vi "teste-Image-2.vi"() -> ()   [LabVIEW 2014]
panel:
  out "size(s) 3":i32=5760000
  out "image":u8[](array[numeric])
  out "size(s) 2":i32=1600
  out "size(s)":i32[](array[numeric])=[1200, 1600]
  out "Waveform Graph":u8[](graph)=[0, 0, 0, 0, 0, 0, 0, 0, 0, 0, 0, 0, 0, 0, 0, 0, 0, 0, 0, 0, 0, 0, 0, 0, 0, 0, 0, 0, 0, 0, 0, 0, 0, 0, 0, 0, 0, 0, 0, 0, 0, 0, 0, 0, 0, 0, 0, 0, 0, 0, 0, 0, 0, 0, 0, 0, 0, 0, 0, 0, 0, 0, 0, 0, 0, 0, 0, 0, 0, 0, 0, 0, 0, 0, 0, 0, 0, 0, 0, 0, 0, 0, 0, 0, 0, 0, 0, 0, 0, 0, 0, 0, 0, 0, 0, 0, 0, 0, 0, 0, 0, 0, 0, 0, 0, 0, 0, 0, 0, 0, 0, 0, 0, 0, 0, 0, 0, 0, 0, 0, 0, 0, 0, 0, 0, 0, 0, 0, 0, 0, 0, 0, 0, 0, 0, 0, 0, 0, 0, 0, 0, 0, 0, 0, 0, 0, 0, 0, 0, 0, 0, 0, 0, 0, 0, 0, 0, 0, 0, 0, 0, 0, 0, 0, 0, 0, 0, 0, 0, 0, 0, 0, 0, 0, 0, 0, 0, 0, 0, 0, 0, 0, 0, 0, 2, 2, 1, 0, 0, 0, 0, 1, 0, 0, 1, 1, 0, 0, 1, 2, 0, 0, 0, 0, 0, 0, 0, 0, 0, 0, 0, 0, 0, 0, 0, 0, 0, 0, 0, 0, 0, 0, 0, 0, 1, 1, 1, 1, 1, 1, 1, 1, 1, 1, 3, 5, 3, 1, 1, 3, 0, 0, 0, 0, 0, 0, 0, 0, 0, 0, 0, 0, 0, 0, 0, 0, 0, 0, 0, 0, 0, 0, 0, 0, 0, 0, 0, 0, 0, 0, 0, 0, 0, 3, 4, 0, 1, 4, 5, 3, 4, 4, 4, 1, 0, 0, 0, 0, 0, 0, 0, 0, 0, 0, 0, 0, 0, 0, 0, 0, 0, 0, 0, 0, 0, 0, 0, 0, 0, 0, 0, 0, 0, 0, 0, 0, 0, 0, 0, 0, 0, 0, 0, 0, 0, 0, 0, 0, 0, 0, 0, 0, 0, 0, 0, 0, 0, 0, 0, 0, 0, 0, 0, 0, 0, 0, 0, 0, 0, 0, 0, 0, 2, 4, 7, 5, 4, 1, 5, 5, 4, 2, 4, 2, 7, 9, 13, 10, 1, 0, 0, 0, 0, 0, 0, 0, 0, 1, 2, 2, 0, 0, 1, 3, 2, 4, 3, 3, 4, 4, 4, 4, 7, 8, 9, 5, 5, 5, 6, 3, 2, 1, 1, 3, 4, 6, 10, 11, 11, 9, 8, 12, 16, 17, 13, 10, 28, 28, 18, 26, 13, 26, 14, 7, 11, 9, 11, 15, 13, 15, 16, 34, 10, 10, 13, 8, 10, 11, 14, 34, 11, 12, 9, 9, 8, 7, 9, 13, 10, 14, 9, 10, 6, 3, 5, 3, 4, 4, 10, 5, 7, 8, 13, 9, 10, 11, 10, 8, 5, 4, 5, 4, 0, 0, 1, 1, 0, 0, 0, 0, 0, 1, 1, 1, 1, 1, 1, 1, 2, 1, 1, 1, 1, 1, 1, 2, 0, 0, 0, 0, 0, 0, 0, 0, 2, 2, 2, 2, 1, 0, 0, 1, 5, 2, 1, 1, 4, 5, 3, 1, 4, 1, 1, 3, 5, 3, 4, 5, 8, 8, 11, 13, 9, 6, 9, 15, 9, 16, 18, 20, 24, 49, 40, 33, 56, 47, 28, 46, 33, 58, 62, 66, 72, 56, 53, 35, 40, 46, 63, 73, 83, 83, 80, 79, 78, 75, 75, 75, 75, 76, 66, 71, 71, 65, 76, 79, 82, 86, 87, 90, 91, 91, 91, 92, 98, 95, 95, 99, 99, 97, 99, 102, 98, 101, 102, 100, 100, 101, 100, 97, 100, 99, 99, 101, 103, 103, 101, 98, 98, 98, 99, 97, 99, 97, 97, 97, 99, 97, 94, 93, 94, 95, 96, 95, 90, 91, 93, 93, 91, 89, 88, 88, 85, 86, 85, 83, 81, 80, 81, 81, 85, 83, 83, 85, 84, 81, 77, 80, 86, 84, 80, 77, 78, 78, 79, 74, 67, 41, 40, 39, 56, 42, 45, 44, 47, 47, 54, 64, 71, 73, 74, 74, 68, 54, 66, 54, 65, 69, 55, 69, 63, 66, 74, 81, 77, 78, 84, 91, 96, 99, 98, 98, 96, 95, 94, 94, 96, 98, 98, 100, 101, 101, 103, 103, 106, 106, 109, 109, 111, 113, 114, 114, 116, 114, 115, 113, 114, 113, 114, 115, 115, 116, 117, 120, 120, 120, 121, 121, 120, 120, 123, 123, 125, 125, 126, 126, 127, 127, 129, 130, 131, 131, 134, 134, 136, 136, 136, 136, 136, 135, 137, 135, 134, 132, 131, 131, 131, 130, 130, 129, 129, 128, 128, 128, 128, 128, 126, 126, 125, 125, 125, 126, 128, 128, 130, 130, 130, 130, 128, 128, 126, 125, 125, 125, 125, 125, 125, 124, 123, 122, 122, 122, 124, 122, 124, 121, 121, 120, 120, 120, 121, 121, 120, 119, 118, 118, 118, 118, 115, 115, 115, 116, 116, 115, 114, 113, 104, 103, 104, 103, 99, 98, 98, 97, 96, 94, 93, 90, 90, 90, 91, 90, 86, 86, 84, 75, 76, 79, 53, 39, 41, 33, 27, 24, 21, 16, 14, 14, 22, 25, 9, 7, 6, 4, 15, 4, 3, 1, 1, 1, 2, 4, 3, 3, 8, 12, 13, 7, 4, 4, 6, 4, 4, 6, 7, 3, 5, 3, 4, 5, 7, 4, 6, 15, 13, 37, 19, 8, 8, 1, 1, 4, 4, 10, 15, 12, 8, 12, 13, 26, 36, 35, 42, 49, 31, 38, 35, 41, 44, 73, 54, 54, 57, 54, 55, 72, 64, 78, 69, 73, 77, 78, 73, 67, 71, 72, 68, 72, 81, 85, 87, 87, 85, 87, 88, 90, 89, 90, 91, 93, 93, 91, 89, 85, 76, 74, 69, 81, 76, 68, 63, 86, 80, 85, 84, 82, 83, 86, 85, 79, 73, 68, 80, 61, 46, 41, 49, 43, 45, 59, 48, 53, 59, 54, 58, 72, 56, 71, 71, 61, 71, 60, 49, 50, 45, 27, 20, 23, 13, 16, 28, 13, 8, 11, 14, 10, 4, 3, 1, 2, 1, 1, 1, 0, 1, 0, 0, 0, 0, 0, 0, 0, 0, 0, 0, 0, 0, 0, 0, 0, 0, 0, 0, 0, 0, 0, 0, 0, 0, 0, 0, 0, 0, 0, 0, 0, 0, 0, 0, 0, 0, 0, 0, 0, 0, 0, 1, 1, 15, 7, 1, 1, 4, 2, 4, 5, 4, 5, 4, 4, 2, 2, 1, 0, 0, 1, 2, 3, 5, 5, 6, 6, 3, 4, 4, 3, 3, 7, 6, 3, 3, 3, 3, 3, 3, 3, 3, 3, 7, 3, 8, 6, 41, 15, 12, 39, 26, 18, 12, 10, 8, 3, 1, 5, 21, 4, 3, 9, 5, 10, 15, 6, 7, 5, 4, 3, 2, 1, 1, 3, 1, 3, 4, 4, 1, 1, 5, 1, 1, 1, 1, 1, 1, 1, 1, 1, 1, 2, 3, 2, 1, 1, 2, 4, 2, 2, 2, 1, 1, 3, 10, 15, 4, 1, 0, 0, 3, 4, 2, 0, 0, 0, 0, 0, 0, 0, 0, 0, 0, 0, 0, 0, 0, 0, 0, 0, 0, 0, 0, 0, 0, 0, 0, 0, 0, 0, 0, 0, 0, 0, 0, 0, 0, 0, 0, 0, 0, 0, 0, 0, 0, 0, 0, 0, 0, 0, 0, 0, 0, 0, 0, 0, 0, 0, 0, 0, 1, 0, 0, 0, 0, 0, 0, 1, 0, 0, 0, 0, 0, 0, 0, 0, 0, 0, 0, 0, 0, 0, 0, 0, 0, 0, 0, 0, 0, 0, 0, 0, 0, 0, 0, 0, 0, 0, 0, 0, 0, 0, 0, 0, 0, 0, 0, 0, 0, 0, 0, 0, 0, 0, 0, 0, 0, 0, 0, 0, 0, 0, 0, 0, 0, 0, 0, 0, 0, 0, 0, 0, 0, 0, 0, 0, 0, 0, 0, 0, 0, 0, 0, 0, 0, 0, 0, 0, 0, 0, 0, 0, 0, 0, 0, 0, 0, 0, 0, 0, 0, 0, 0, 0, 0, 0, 0, 0, 0, 0, 0, 0, 0, 0, 0, 0, 0, 0, 0, 0, 0, 0, 0, 0, 0, 0, 0, 0, 0, 0, 0, 0, 0, 0, 0, 0, 0, 0, 0, 0, 0, 0, 0, 0, 0, 0, 0, 0, 0, 0, 0, 0, 0, 0, 0, 0, 0, 0, 0, 0, 0, 0, 0, 0, 0, 0, 0, 0, 0, 0, 0, 0, 0, 0, 0, 0, 0, 0, 0, 0, 0, 0, 0, 0, 0, 0, 0, 0, 0, 0, 0, 0, 0, 0, 0, 0, 0, 0, 0, 0, 0, 0, 0, 0, 0, 0, 0, 0, 0, 0, 0, 0, 0, 0, 0, 0, 0, 0, 0, 0, 0, 0, 0, 0, 0, 0, 0, 0, 0, 0, 0, 0, 0, 0, 0, 0, 0, 0, 0, 0, 1, 0, 0, 0, 0, 0, 0, 1, 0, 0, 0, 0, 0, 0, 0, 0, 0, 0, 0, 0, 0, 0, 0, 0, 0, 0, 0, 0, 0, 0, 0, 0, 0, 0, 0, 0, 0, 0, 0, 0, 0, 0, 0, 0, 0, 0, 0, 0, 0, 0, 0, 0, 0, 0, 0, 0, 0, 0, 0, 0, 0, 0, 0, 0, 0, 0, 0, 0, 0, 0, 0, 0, 0, 0, 0, 0, 0, 0, 0, 0, 0, 0, 0, 0, 0, 0, 0, 0, 0, 0, 0, 0, 0, 0, 0, 0, 0, 0, 0, 0, 0, 0, 0, 0, 0, 0, 0, 0, 0, 0, 0, 0, 0, 0, 2, 4, 4, 2, 0, 0, 0, 0, 0, 0, 0, 0, 0, 0, 0, 0, 0, 0, 0, 0, 0, 0, 0, 0, 0, 0, 0, 0, 0, 0]
  out "2D Picture":picture
  out "subarray":u8[](array[numeric])=[0, 0, 0, 0, 0, 0, 0, 0, 0, 0, 0, 0, 0, 0, 0, 0, 0, 0, 0, 0, 0, 0, 0, 0, 0, 0, 0, 0, 0, 0, 0, 0, 0, 0, 0, 0, 0, 0, 0, 0, 0, 0, 0, 0, 0, 0, 0, 0, 0, 0, 0, 0, 0, 0, 0, 0, 0, 0, 0, 0, 0, 0, 0, 0, 0, 0, 0, 0, 0, 0, 0, 0, 0, 0, 0, 0, 0, 0, 0, 0, 0, 0, 0, 0, 0, 0, 0, 0, 0, 0, 0, 0, 0, 0, 0, 0, 0, 0, 0, 0, 0, 0, 0, 0, 0, 0, 0, 0, 0, 0, 0, 0, 0, 0, 0, 0, 0, 0, 0, 0, 0, 0, 0, 0, 0, 0, 0, 0, 0, 0, 0, 0, 0, 0, 0, 0, 0, 0, 0, 0, 0, 0, 0, 0, 0, 0, 0, 0, 0, 0, 0, 0, 0, 0, 0, 0, 0, 0, 0, 0, 0, 0, 0, 0, 0, 0, 0, 0, 0, 0, 0, 0, 0, 0, 0, 0, 0, 0, 0, 0, 0, 0, 0, 0, 2, 2, 1, 0, 0, 0, 0, 1, 0, 0, 1, 1, 0, 0, 1, 2, 0, 0, 0, 0, 0, 0, 0, 0, 0, 0, 0, 0, 0, 0, 0, 0, 0, 0, 0, 0, 0, 0, 0, 0, 1, 1, 1, 1, 1, 1, 1, 1, 1, 1, 3, 5, 3, 1, 1, 3, 0, 0, 0, 0, 0, 0, 0, 0, 0, 0, 0, 0, 0, 0, 0, 0, 0, 0, 0, 0, 0, 0, 0, 0, 0, 0, 0, 0, 0, 0, 0, 0, 0, 3, 4, 0, 1, 4, 5, 3, 4, 4, 4, 1, 0, 0, 0, 0, 0, 0, 0, 0, 0, 0, 0, 0, 0, 0, 0, 0, 0, 0, 0, 0, 0, 0, 0, 0, 0, 0, 0, 0, 0, 0, 0, 0, 0, 0, 0, 0, 0, 0, 0, 0, 0, 0, 0, 0, 0, 0, 0, 0, 0, 0, 0, 0, 0, 0, 0, 0, 0, 0, 0, 0, 0, 0, 0, 0, 0, 0, 0, 0, 2, 4, 7, 5, 4, 1, 5, 5, 4, 2, 4, 2, 7, 9, 13, 10, 1, 0, 0, 0, 0, 0, 0, 0, 0, 1, 2, 2, 0, 0, 1, 3, 2, 4, 3, 3, 4, 4, 4, 4, 7, 8, 9, 5, 5, 5, 6, 3, 2, 1, 1, 3, 4, 6, 10, 11, 11, 9, 8, 12, 16, 17, 13, 10, 28, 28, 18, 26, 13, 26, 14, 7, 11, 9, 11, 15, 13, 15, 16, 34, 10, 10, 13, 8, 10, 11, 14, 34, 11, 12, 9, 9, 8, 7, 9, 13, 10, 14, 9, 10, 6, 3, 5, 3, 4, 4, 10, 5, 7, 8, 13, 9, 10, 11, 10, 8, 5, 4, 5, 4, 0, 0, 1, 1, 0, 0, 0, 0, 0, 1, 1, 1, 1, 1, 1, 1, 2, 1, 1, 1, 1, 1, 1, 2, 0, 0, 0, 0, 0, 0, 0, 0, 2, 2, 2, 2, 1, 0, 0, 1, 5, 2, 1, 1, 4, 5, 3, 1, 4, 1, 1, 3, 5, 3, 4, 5, 8, 8, 11, 13, 9, 6, 9, 15, 9, 16, 18, 20, 24, 49, 40, 33, 56, 47, 28, 46, 33, 58, 62, 66, 72, 56, 53, 35, 40, 46, 63, 73, 83, 83, 80, 79, 78, 75, 75, 75, 75, 76, 66, 71, 71, 65, 76, 79, 82, 86, 87, 90, 91, 91, 91, 92, 98, 95, 95, 99, 99, 97, 99, 102, 98, 101, 102, 100, 100, 101, 100, 97, 100, 99, 99, 101, 103, 103, 101, 98, 98, 98, 99, 97, 99, 97, 97, 97, 99, 97, 94, 93, 94, 95, 96, 95, 90, 91, 93, 93, 91, 89, 88, 88, 85, 86, 85, 83, 81, 80, 81, 81, 85, 83, 83, 85, 84, 81, 77, 80, 86, 84, 80, 77, 78, 78, 79, 74, 67, 41, 40, 39, 56, 42, 45, 44, 47, 47, 54, 64, 71, 73, 74, 74, 68, 54, 66, 54, 65, 69, 55, 69, 63, 66, 74, 81, 77, 78, 84, 91, 96, 99, 98, 98, 96, 95, 94, 94, 96, 98, 98, 100, 101, 101, 103, 103, 106, 106, 109, 109, 111, 113, 114, 114, 116, 114, 115, 113, 114, 113, 114, 115, 115, 116, 117, 120, 120, 120, 121, 121, 120, 120, 123, 123, 125, 125, 126, 126, 127, 127, 129, 130, 131, 131, 134, 134, 136, 136, 136, 136, 136, 135, 137, 135, 134, 132, 131, 131, 131, 130, 130, 129, 129, 128, 128, 128, 128, 128, 126, 126, 125, 125, 125, 126, 128, 128, 130, 130, 130, 130, 128, 128, 126, 125, 125, 125, 125, 125, 125, 124, 123, 122, 122, 122, 124, 122, 124, 121, 121, 120, 120, 120, 121, 121, 120, 119, 118, 118, 118, 118, 115, 115, 115, 116, 116, 115, 114, 113, 104, 103, 104, 103, 99, 98, 98, 97, 96, 94, 93, 90, 90, 90, 91, 90, 86, 86, 84, 75, 76, 79, 53, 39, 41, 33, 27, 24, 21, 16, 14, 14, 22, 25, 9, 7, 6, 4, 15, 4, 3, 1, 1, 1, 2, 4, 3, 3, 8, 12, 13, 7, 4, 4, 6, 4, 4, 6, 7, 3, 5, 3, 4, 5, 7, 4, 6, 15, 13, 37, 19, 8, 8, 1, 1, 4, 4, 10, 15, 12, 8, 12, 13, 26, 36, 35, 42, 49, 31, 38, 35, 41, 44, 73, 54, 54, 57, 54, 55, 72, 64, 78, 69, 73, 77, 78, 73, 67, 71, 72, 68, 72, 81, 85, 87, 87, 85, 87, 88, 90, 89, 90, 91, 93, 93, 91, 89, 85, 76, 74, 69, 81, 76, 68, 63, 86, 80, 85, 84, 82, 83, 86, 85, 79, 73, 68, 80, 61, 46, 41, 49, 43, 45, 59, 48, 53, 59, 54, 58, 72, 56, 71, 71, 61, 71, 60, 49, 50, 45, 27, 20, 23, 13, 16, 28, 13, 8, 11, 14, 10, 4, 3, 1, 2, 1, 1, 1, 0, 1, 0, 0, 0, 0, 0, 0, 0, 0, 0, 0, 0, 0, 0, 0, 0, 0, 0, 0, 0, 0, 0, 0, 0, 0, 0, 0, 0, 0, 0, 0, 0, 0, 0, 0, 0, 0, 0, 0, 0, 0, 0, 1, 1, 15, 7, 1, 1, 4, 2, 4, 5, 4, 5, 4, 4, 2, 2, 1, 0, 0, 1, 2, 3, 5, 5, 6, 6, 3, 4, 4, 3, 3, 7, 6, 3, 3, 3, 3, 3, 3, 3, 3, 3, 7, 3, 8, 6, 41, 15, 12, 39, 26, 18, 12, 10, 8, 3, 1, 5, 21, 4, 3, 9, 5, 10, 15, 6, 7, 5, 4, 3, 2, 1, 1, 3, 1, 3, 4, 4, 1, 1, 5, 1, 1, 1, 1, 1, 1, 1, 1, 1, 1, 2, 3, 2, 1, 1, 2, 4, 2, 2, 2, 1, 1, 3, 10, 15, 4, 1, 0, 0, 3, 4, 2, 0, 0, 0, 0, 0, 0, 0, 0, 0, 0, 0, 0, 0, 0, 0, 0, 0, 0, 0, 0, 0, 0, 0, 0, 0, 0, 0, 0, 0, 0, 0, 0, 0, 0, 0, 0, 0, 0, 0, 0, 0, 0, 0, 0, 0, 0, 0, 0, 0, 0, 0, 0, 0, 0, 0, 0, 0, 1, 0, 0, 0, 0, 0, 0, 1, 0, 0, 0, 0, 0, 0, 0, 0, 0, 0, 0, 0, 0, 0, 0, 0, 0, 0, 0, 0, 0, 0, 0, 0, 0, 0, 0, 0, 0, 0, 0, 0, 0, 0, 0, 0, 0, 0, 0, 0, 0, 0, 0, 0, 0, 0, 0, 0, 0, 0, 0, 0, 0, 0, 0, 0, 0, 0, 0, 0, 0, 0, 0, 0, 0, 0, 0, 0, 0, 0, 0, 0, 0, 0, 0, 0, 0, 0, 0, 0, 0, 0, 0, 0, 0, 0, 0, 0, 0, 0, 0, 0, 0, 0, 0, 0, 0, 0, 0, 0, 0, 0, 0, 0, 0, 0, 0, 0, 0, 0, 0, 0, 0, 0, 0, 0, 0, 0, 0, 0, 0, 0, 0, 0, 0, 0, 0, 0, 0, 0, 0, 0, 0, 0, 0, 0, 0, 0, 0, 0, 0, 0, 0, 0, 0, 0, 0, 0, 0, 0, 0, 0, 0, 0, 0, 0, 0, 0, 0, 0, 0, 0, 0, 0, 0, 0, 0, 0, 0, 0, 0, 0, 0, 0, 0, 0, 0, 0, 0, 0, 0, 0, 0, 0, 0, 0, 0, 0, 0, 0, 0, 0, 0, 0, 0, 0, 0, 0, 0, 0, 0, 0, 0, 0, 0, 0, 0, 0, 0, 0, 0, 0, 0, 0, 0, 0, 0, 0, 0, 0, 0, 0, 0, 0, 0, 0, 0, 0, 0, 0, 0, 0, 1, 0, 0, 0, 0, 0, 0, 1, 0, 0, 0, 0, 0, 0, 0, 0, 0, 0, 0, 0, 0, 0, 0, 0, 0, 0, 0, 0, 0, 0, 0, 0, 0, 0, 0, 0, 0, 0, 0, 0, 0, 0, 0, 0, 0, 0, 0, 0, 0, 0, 0, 0, 0, 0, 0, 0, 0, 0, 0, 0, 0, 0, 0, 0, 0, 0, 0, 0, 0, 0, 0, 0, 0, 0, 0, 0, 0, 0, 0, 0, 0, 0, 0, 0, 0, 0, 0, 0, 0, 0, 0, 0, 0, 0, 0, 0, 0, 0, 0, 0, 0, 0, 0, 0, 0, 0, 0, 0, 0, 0, 0, 0, 0, 0, 2, 4, 4, 2, 0, 0, 0, 0, 0, 0, 0, 0, 0, 0, 0, 0, 0, 0, 0, 0, 0, 0, 0, 0, 0, 0, 0, 0, 0, 0]
  in  "index (row)":i32(slide)=495
  in  "FROG path":path=path "C:/FROG/2022-05-26_10-35-10_RawData-2.jpg"
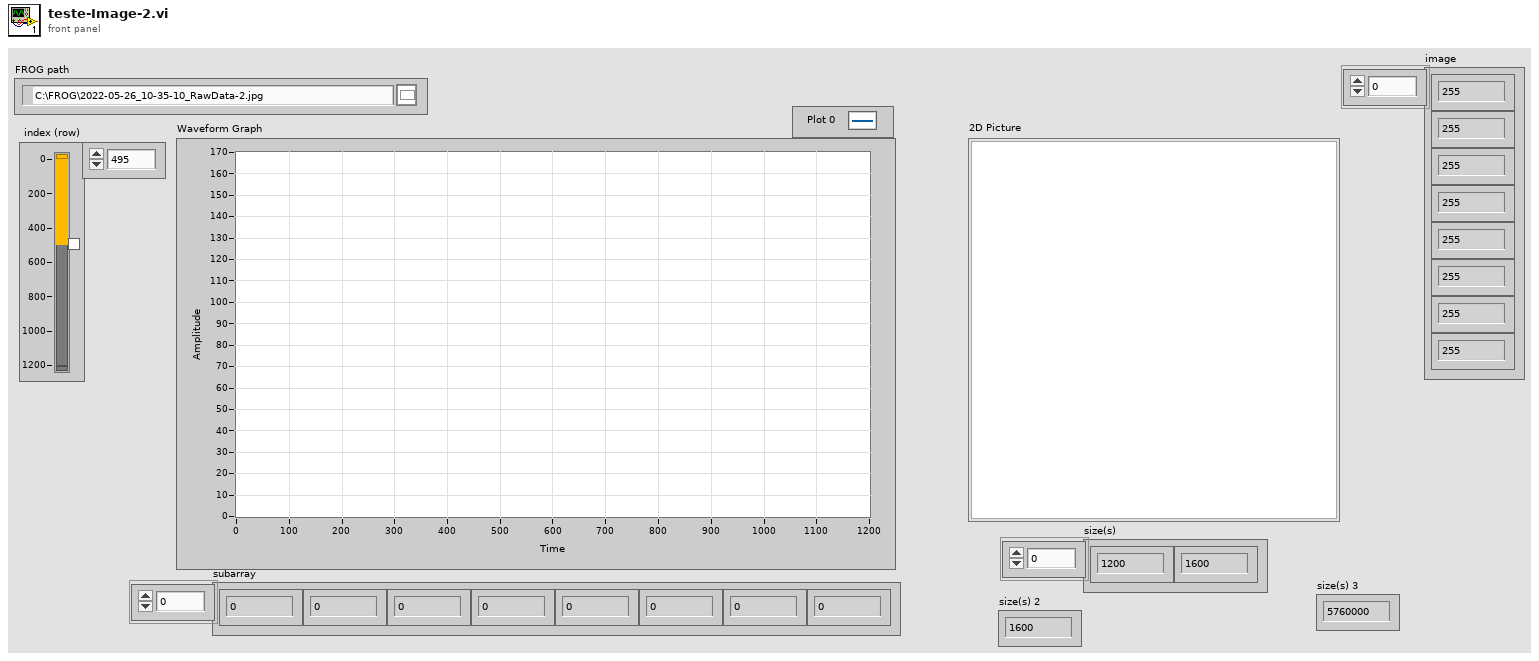
[diagram p1: front panel]
types:
  T1 = typedef "imagedata.ctl" = cluster{"image type":i32, "image depth":i32, "image":u8[], "mask":u8[], "colors":u32[], "Rectangle":cluster{"left":i16, "top":i16, "right":i16, "bottom":i16}}
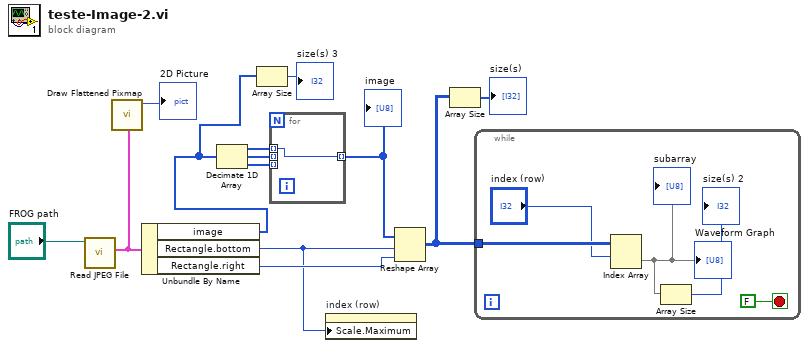
[diagram p0: block diagram]
diagram:
  n1 = call <vilib>:"Read JPEG File.vi"("path to JPEG file"="FROG path") -> ("image data"=w11:T1)  [unwired: 8 in, 2 out]
  n2 = call <vilib>:"Draw Flattened Pixmap.vi"("image data"=w11) -> ("new picture"=→"2D Picture":picture)  [unwired: 8 in]
  n3 = Unbundle By Name(w11) -> ("image"=w4:u8[], "Rectangle.bottom"=w1:i16, "Rectangle.right"=w2:i16)
  n4 = Decimate 1D Array(w4) -> (w8:u8[], w7:u8[], w6:u8[])
  n5 = Array Size(array=w4) -> (size(s)=→"size(s) 3":i32)
  n6 = for {
    tunnel: w8 -> [w14] mode=indexing
    tunnel: w7 -> [_] mode=indexing
    tunnel: w6 -> [_] mode=indexing
    tunnel: [w14] -> w5 mode=indexing
  }
  "image" <- w5
  n7 = property on="index (row)" class="Slide (strict)"("Scale.Maximum"=w1) -> ()  [unwired: 2 in, 2 out]
  n8 = Reshape Array(w5, w1, w2) -> (w10:u8[][])
  n9 = Array Size(array=w10) -> (size(s)=→"size(s)":i32[])
  n10 = while {
    tunnel: w10 -> [w16]
    stop <- FALSE stop-if-true
    n11 = Index Array(array=w16, index (row)="index (row)") -> (element=w18:u8[])  [unwired: 1 in]
    "subarray" <- w18
    "Waveform Graph" <- w18
    n12 = Array Size(array=w18) -> (size(s)=→"size(s) 2":i32)
  }
